vi "setState.vi"(8 "error in (no error)":errorcluster, 9 "Argument":string, 10 "Command":T1=enum."start", 11 "DAQmx in":refnum<class "DAQmx.lvclass">) -> (0 "error out":errorcluster, 3 "DAQmx out":refnum<class "DAQmx.lvclass">)   [LabVIEW 2019, in "DAQmx.lvclass"]
uses:
  DAQmx.lvclass
  typedefs/DAQmx.Commands--enum.ctl
  DAQmx.lvclass/DAQmx.ctl
  typedefs/Message--Cluster.ctl
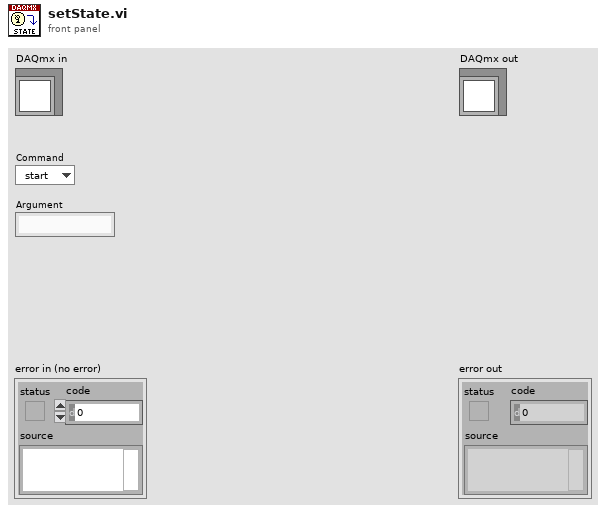
[diagram p1: front panel]
types:
  T1 = typedef "DAQmx.lvclass/DAQmx.Commands--enum.ctl" = enum16{"idle", "start", "stop", "calibrate", "auto", "exit"}
  T2 = typedef "DAQmx.lvclass/Message--Cluster.ctl" = cluster{"command":T1, "Argument":string}
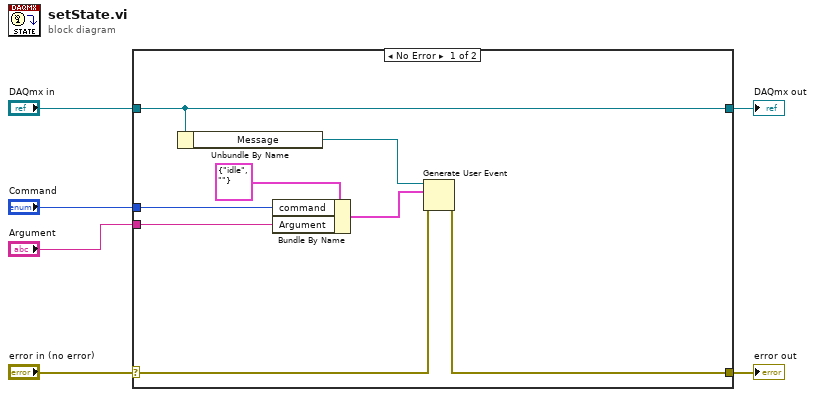
[diagram p0: block diagram]
diagram:
  n1 = case shown="No Error" "error in (no error)" {
    selector: "error in (no error)" -> [w12 w16]
    tunnel: [w11 w16] -> w5
    tunnel: [w14 w15] -> w3
    tunnel: "DAQmx in" -> [w14 w15]
    tunnel: "Command" -> [w9 _]
    tunnel: "Argument" -> [w7 _]
    frame No Error {
      n2 = Unbundle By Name(w14) -> ("Message"=w13:refnum<user-event>)
      n3 = Bundle By Name(cluster=T2 {"command"=enum."idle", "Argument"=""} ("Message"), "command"=w9, "Argument"=w7) -> (w8:T2)
      n4 = Generate User Event(user event=w13, event data cluster=w8, error in=w12) -> (error out=w11:errorcluster)  [unwired: 1 in, 1 out]
    }
    frame Error {
    }
  }
  "error out" <- w5
  "DAQmx out" <- w3
